vi "Parse Errors From Answer.vi"(8 "error in (no error)":errorcluster, 11 "JSON command":string) -> (0 "error out":errorcluster, 1 "key-value pair found?":bool, 2 "isErrorFree?":bool, 3 "formatted error array":string[](array[string]), 4 "decoded JSON-response":string)   [LabVIEW 2023, in "Communicator.lvclass"]
uses:
  Communicator.lvclass
  <vilib>/JDP Science/JSONtext/Next JSON Value.vi
  <vilib>/JDP Science/JSONtext/String Subset.vi
  <vilib>/JDP Science/JSONtext/Parsing/Advance past next JSON Value (inlined COPY).vi
  <vilib>/JDP Science/JSONtext/Parsing/Advance past whitespace.vi
  <vilib>/JDP Science/JSONtext/Parsing/Advance past String.vi
  <vilib>/JDP Science/JSONtext/Parsing/Advance past Number.vi
  <vilib>/JDP Science/JSONtext/Parsing/Advance past Line Ending.vi
  <vilib>/JDP Science/JSONtext/Parsing/Parse Full Path or Item Name.vi
  <vilib>/JDP Science/JSONtext/Parsing/Advance past Array.vi
  <vilib>/JDP Science/JSONtext/Parsing/Advance past Object.vi
  <vilib>/JDP Science/JSONtext/support/Error Cluster From Code.vi
  <vilib>/JDP Science/JSONtext/Offset/Find Item Locations by Path.vi
  <vilib>/JDP Science/JSONtext/JSONtext.lvlib
panel:
  # "Connector Pane"
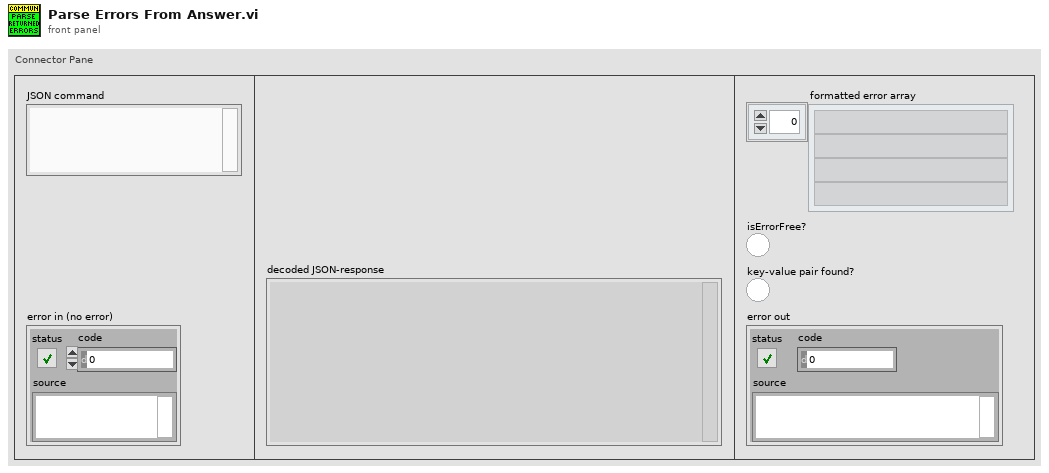
[diagram p1: front panel]
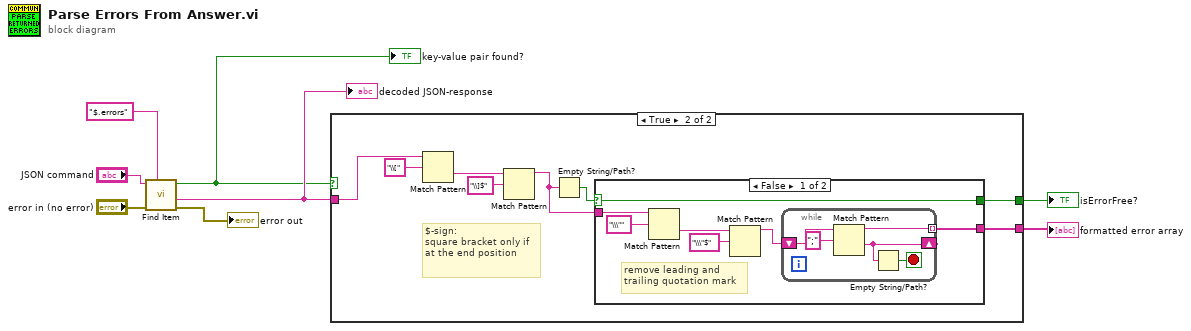
[diagram p0: block diagram]
diagram:
  n1 = call <vilib>:"Find Item.vi"("$Path or Item Name"="$.errors", "error in (no error)"="error in (no error)", "JSON"="JSON command") -> ("error out"=→"error out":errorcluster, "<JSON>"=w5:string, "Found"=w1:bool)  [unwired: 5 in, 1 out]
  "decoded JSON-response" <- w5
  "key-value pair found?" <- w1
  n2 = case shown="True" w1 {
    selector: w1 -> [w9 _]
    tunnel: w5 -> [_ w16]
    tunnel: [w9 w12] -> w2
    tunnel: [_ w10] -> w3
    frame False {
    }
    frame True {
      # "$-sign:\nsquare bracket only if at the end position"
      n3 = Match Pattern(string=w16, regular expression="\\[" ("$Path or Item Name")) -> (after substring=w15:string)  [unwired: 1 in, 3 out]
      n4 = Match Pattern(string=w15, regular expression="\\]$" ("$Path or Item Name")) -> (before substring=w11:string)  [unwired: 1 in, 3 out]
      n5 = Empty String/Path?(string/path=w11) -> (empty?=w13:bool)
      n6 = case shown="False" w13 {
        selector: w13 -> [w23 w30]
        tunnel: [w23 w30] -> w12
        tunnel: w11 -> [w19 _]
        tunnel: [w24 _] -> w10
        frame False {
          # "remove leading and\ntrailing quotation mark"
          n7 = Match Pattern(string=w19, regular expression="\\\"" ("$Path or Item Name")) -> (after substring=w21:string)  [unwired: 1 in, 3 out]
          n8 = Match Pattern(string=w21, regular expression="\\\"$" ("$Path or Item Name")) -> (before substring=w18:string)  [unwired: 1 in, 3 out]
          n9 = while {
            tunnel: [w27] -> w24 mode=indexing
            shift-right: [w26] -> _
            shift-left: w18 -> [w28]
            stop <- w25 stop-if-true
            n10 = Match Pattern(string=w28, regular expression=";") -> (before substring=w27:string, after substring=w26:string)  [unwired: 1 in, 2 out]
            n11 = Empty String/Path?(string/path=w26) -> (empty?=w25:bool)
          }
        }
        frame True {
          # "error string empty"
        }
      }
    }
  }
  "formatted error array" <- w3
  "isErrorFree?" <- w2
